vi "Output Sound Tone till acq complete.vi"(0 "device ID":u32, 1 "frequency":dbl=500.0 format="%0.2p", 2 "volume":dbl(slide)=100.0 min=0.0 max=100.0 step=1.0 scale=0.0..100.0) -> (7 "error out":errorcluster)   [LabVIEW 2022 SP3]
uses:
  <vilib>/sound2/lvsound2.llb/Sound Data Format.ctl
  <vilib>/sound2/lvsound2.llb/Sampling Mode.ctl
  Anemometry/Anemometry Sub Vis/Globals/Meas_global.vi
  <vilib>/sound2/lvsound2.llb/Sound Output Set Volume (Single).vi
  <vilib>/sound2/lvsound2.llb/Sound Output Write (DBL).vi
  <vilib>/measure/NI_MABase.lvlib
panel:
  in  "stop":bool
  out "loop":i32
  in  "sound format":T1={"sample rate (S/s)"=44100.0, "number of channels"=2, "bits per sample"=16}
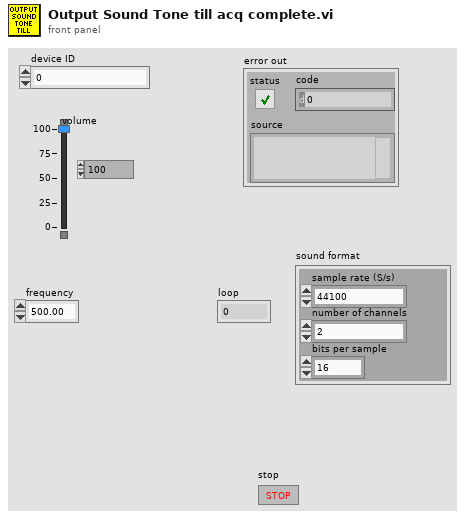
[diagram p1: front panel]
types:
  T1 = typedef "Sound Data Format.ctl" = cluster{"sample rate (S/s)":dbl, "number of channels":i32, "bits per sample":i32}
  T2 = typedef "Sampling Mode.ctl" = i32
  T3 = typedef "Sound Output Task ID.ctl" = u32
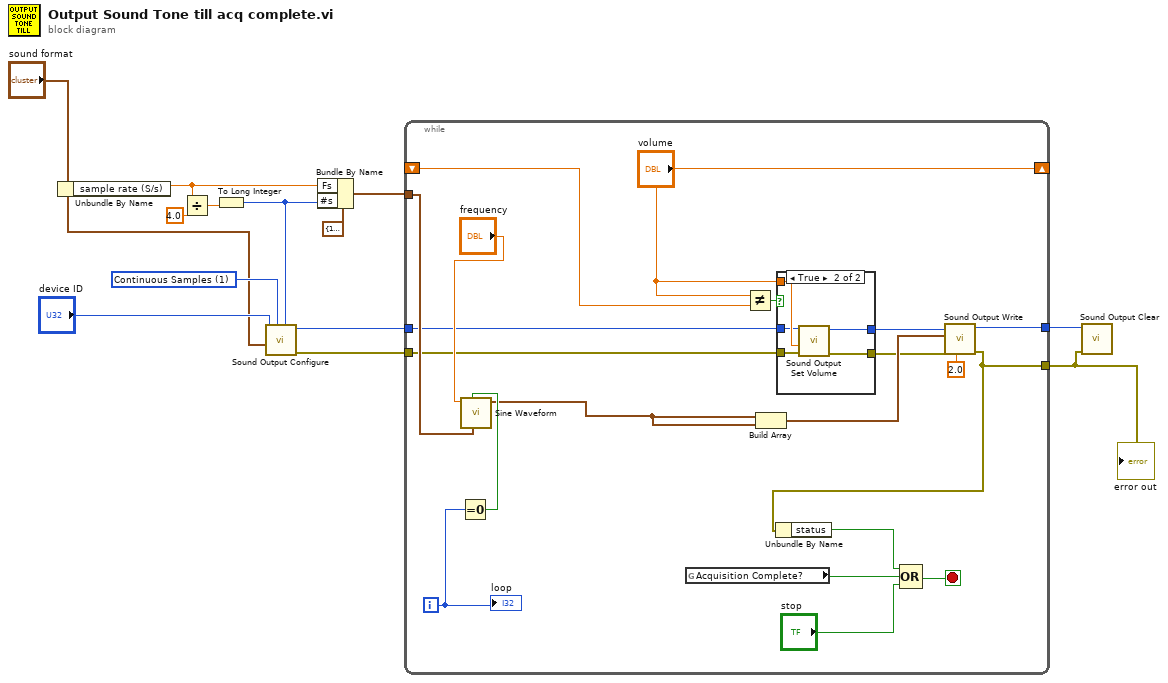
[diagram p0: block diagram]
diagram:
  w12 = T2 1 items=["Finite Samples", "Continuous Samples"] ("sample mode")
  n1 = Unbundle By Name("sound format") -> ("sample rate (S/s)"=w4:dbl)
  n2 = Divide(x=w4, y=4.0) -> (x/y=w8:dbl)
  n3 = To Long Integer(number=w8) -> (32bit integer=w2:i32)
  n4 = call <vilib>:"Sound Output Configure.vi"("number of samples/ch"=w2, "sample mode"=w12, "sound format"="sound format", "device ID"="device ID") -> ("error out"=w6:errorcluster, "task ID"=w13:T3)  [unwired: 6 in]
  n5 = Bundle By Name(cluster=cluster{"Fs":dbl, "#s":dbl} {"Fs"=1000.0, "#s"=1000.0} ("sampling info"), "Fs"=w4, "#s"=w2) -> (w3:cluster{"Fs":dbl, "#s":dbl})
  n6 = while {
    tunnel: w13 -> [w27]
    tunnel: [w33] -> w7
    tunnel: w6 -> [w25]
    tunnel: w3 -> [w30]
    shift-right: ["volume"] -> _
    shift-left: _ -> [w23]
    tunnel: [w18] -> w1
    i -> [w19]
    stop <- w14 stop-if-true
    n7 = Equal To 0?(x=w19) -> (x = 0?=w32:bool)
    n8 = call <vilib>:"Sine Waveform.vi"("sampling info"=w30, "reset signal"=w32, "frequency"="frequency") -> ("signal out"=w20:waveform(dbl))  [unwired: 7 in, 1 out]
    n9 = global read "Meas_global.vi" "Acquisition Complete?"() -> (w16:bool)
    n10 = Not Equal?(x="volume", y=w23) -> (x != y?=w21:bool)
    n11 = Build Array(w20, w20) -> (w31:waveform(dbl)[])
    n12 = case shown="True" w21 {
      tunnel: "volume" -> [_ w40]
      tunnel: w27 -> [w35 w39]
      tunnel: [w35 w38] -> w26
      tunnel: w25 -> [w34 w37]
      tunnel: [w34 w36] -> w24
      frame False {
      }
      frame True {
        n13 = call-poly <vilib>:"Sound Output Set Volume.vi"("error in (no error)"=w37, "volume"=w40, "task ID"=w39) -> ("error out"=w36:errorcluster, "task ID out"=w38:T3)  [unwired: 7 in]
      }
    }
    n14 = call-poly <vilib>:"Sound Output Write.vi"("timeout (sec)"=2.0, "error in (no error)"=w24, "data"=w31, "task ID"=w26) -> ("error out"=w18:errorcluster, "task ID out"=w33:T3)  [unwired: 6 in]
    n15 = Unbundle By Name(w18) -> ("status"=w17:bool)
    n16 = Compound Arithmetic op=OR(w17, w16, "stop") -> (w14:bool)
    "loop" <- w19
  }
  "error out" <- w1
  n17 = call <vilib>:"Sound Output Clear.vi"("error in (no error)"=w1, "task ID"=w7) -> ()  [unwired: 9 in, 1 out]
